vi "helloworld.vi"() -> ()   [LabVIEW 2020]
panel:
  out "Gauge":dbl(knob) scale=0.0..10.0
  in  "Dial 2":dbl(knob) scale=0.0..10.0
  in  "Dial":dbl(knob) scale=0.0..10.0
  out "String":string
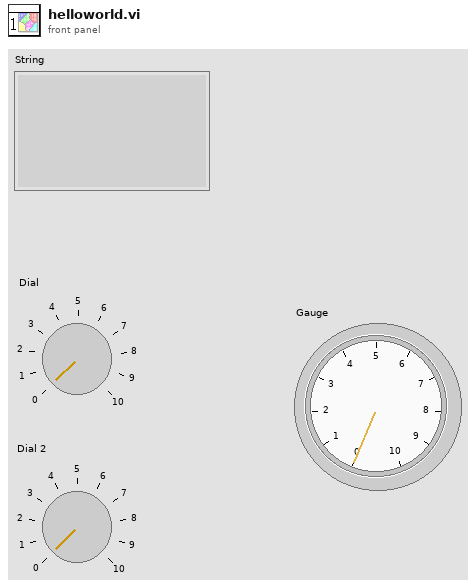
[diagram p1: front panel]
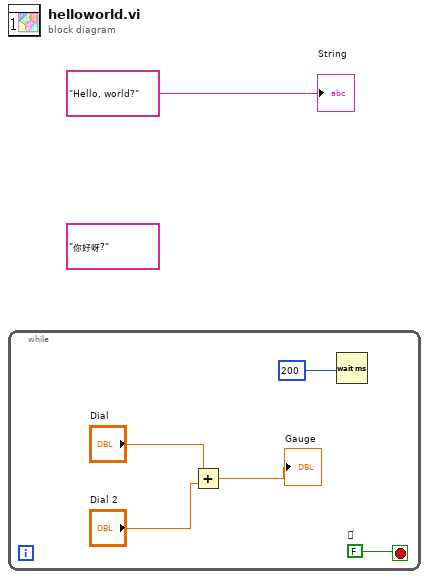
[diagram p0: block diagram]
diagram:
  (unwired) "你好呀?"
  n1 = while {
    stop <- w2 stop-if-true
    w2 = FALSE  # ֹͣ
    n2 = Add(x="Dial", y="Dial 2") -> (x+y=→"Gauge":dbl)
    n3 = Wait (ms)(milliseconds to wait=200) -> ()  [unwired: 1 out]
  }
  "String" <- "Hello, world?"
